vi "Get Vout from Data Out and V Ref.vi"(10 "Vref":dbl=-1.0 format="%.3f V", 11 "Data out (14-bit)":u16 format="%04x") -> (3 "Vout (V)":dbl format="%.3f V")   [LabVIEW 2017, in "Host SRL.lvlib"]
uses:
  Host SRL.lvlib
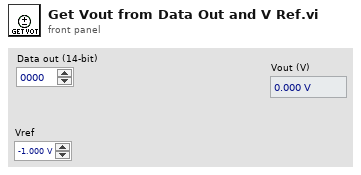
[diagram p1: front panel]
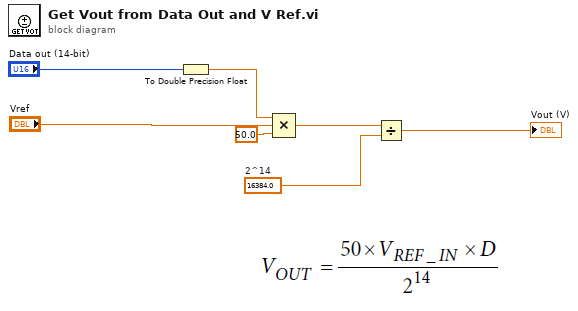
[diagram p0: block diagram]
diagram:
  w2 = 16384.0  # 2^14
  n1 = To Double Precision Float(number="Data out (14-bit)") -> (double precision float=w4:dbl)
  n2 = Compound Arithmetic op=MULTIPLY(w4, "Vref", 50.0 ("y")) -> (w3:dbl)
  n3 = Divide(x=w3, y=w2) -> (x/y=→"Vout (V)":dbl)
